vi "Custom Error Popup.vi"(7 "Message Box":refnum<vi>, 8 "error in (no error)":errorcluster) -> (0 "error out":errorcluster)   [LabVIEW 2014]
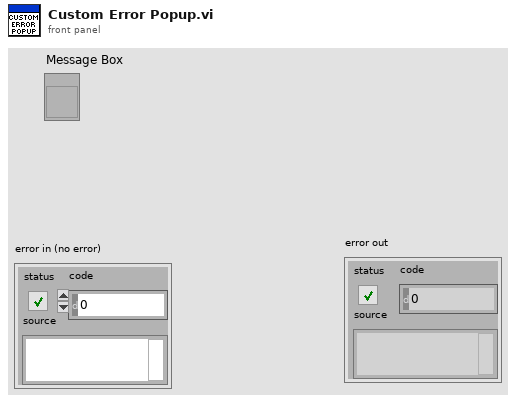
[diagram p1: front panel]
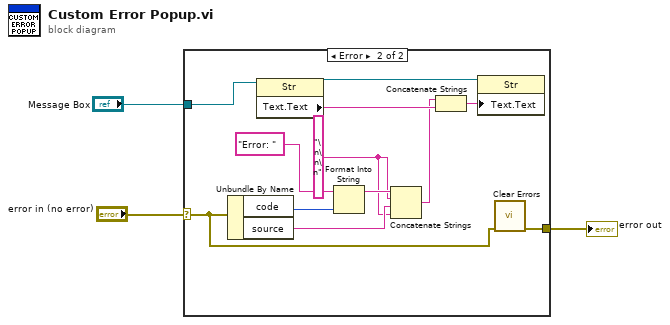
[diagram p0: block diagram]
diagram:
  n1 = case shown="Error" "error in (no error)" {
    selector: "error in (no error)" -> [w4 w12]
    tunnel: [w4 w11] -> w2
    tunnel: "Message Box" -> [_ w10]
    frame No Error {
    }
    frame Error {
      w5 = "\n\n\n" ("string")
      n2 = Unbundle By Name(w12) -> ("code"=w16:i32, "source"=w13:string)
      n3 = property class="Str"(reference=w10) -> (reference out=w6:refnum<vi>, "Text.Text"=w9:string)  [unwired: 1 in, 1 out]
      n4 = Format Into String(initial string="Error: ", w16) -> (resulting string=w14:string)  [unwired: 2 in, 1 out]
      n5 = Concatenate Strings(w14, w5, w13, w5) -> (w8:string)
      n6 = Concatenate Strings(w8, w9) -> (w7:string)
      n7 = property class="Str"(reference=w6, "Text.Text"=w7) -> ()  [unwired: 1 in, 2 out]
      n8 = call <vilib>:"Clear Errors.vi"("error in (no error)"=w12) -> ("error out"=w11:errorcluster)  [unwired: 5 in, 1 out]
    }
  }
  "error out" <- w2
